vi "Write Default Values.vi"(8 "error in (no error)":errorcluster, 10 "Default Values":T1[](array[typedef]), 11 "Toggle 8 in":refnum<class "Toggle 8.lvclass">) -> (0 "error out":errorcluster, 3 "Toggle 8 out":refnum<class "Toggle 8.lvclass">)   [LabVIEW 2020, in "Toggle 8.lvclass"]
uses:
  Toggle 8.lvclass
  Controls/Register to Write.ctl
  Toggle 8.lvclass/Toggle 8.ctl
  PIC-device/PIC-Device.lvclass
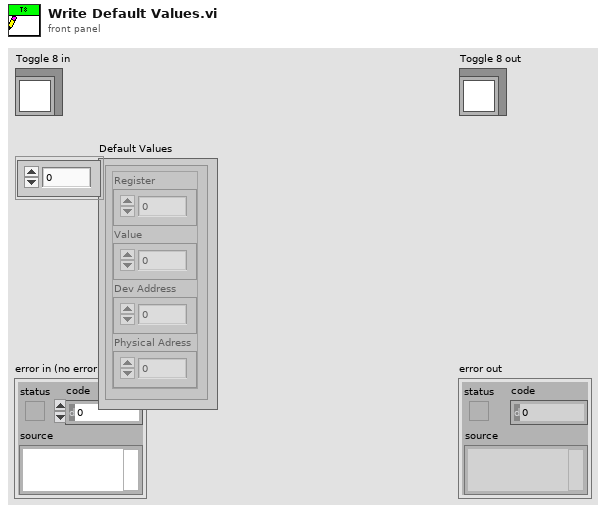
[diagram p1: front panel]
types:
  T1 = typedef "PIC-Device.lvclass/Register to Write.ctl" = cluster{"Register":u32, "Value":u32, "Dev Address":u32, "Physical Adress":u32}
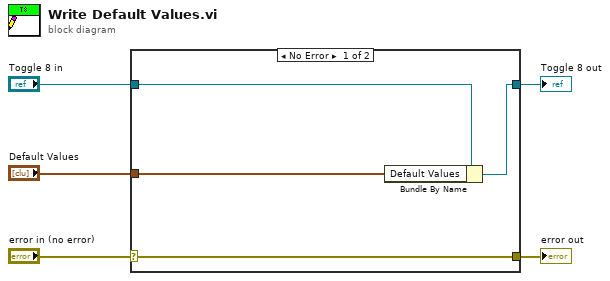
[diagram p0: block diagram]
diagram:
  n1 = case shown="No Error" "error in (no error)" {
    selector: "error in (no error)" -> [w9 w10]
    tunnel: [w9 w10] -> w4
    tunnel: [w7 w11] -> w2
    tunnel: "Toggle 8 in" -> [w8 w11]
    tunnel: "Default Values" -> [w6 _]
    frame No Error {
      n2 = Bundle By Name(cluster=w8, "Default Values"=w6) -> (w7:refnum<class "Toggle 8.lvclass">)
    }
    frame Error {
    }
  }
  "error out" <- w4
  "Toggle 8 out" <- w2
